vi "WriteRead I2C.vi"(5 "Address":u8, 6 "NoStop (F)":bool, 7 "Bus":u8, 8 "error in (no error)":errorcluster, 9 "Read Len":u8, 10 "Write Data":string, 11 "VISA resource name in":refnum<visa-resource-name>) -> (0 "error out":errorcluster, 1 "Read Data":string, 3 "VISA resource name":refnum<visa-resource-name>)   [LabVIEW 2020, in "CTI-Visa.lvlib"]
uses:
  CTI-Visa.lvlib
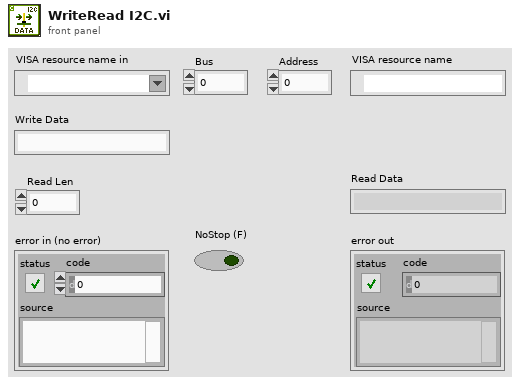
[diagram p1: front panel]
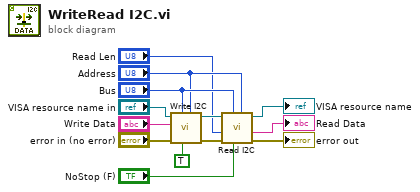
[diagram p0: block diagram]
diagram:
  n1 = call "Write I2C.vi"("Address"="Address", "NoStop (F)"=TRUE, "Bus"="Bus", "error in (no error)"="error in (no error)", "Data"="Write Data", "VISA resource name in"="VISA resource name in") -> ("error out"=w9:errorcluster, "VISA resource name"=w7:refnum<visa-resource-name>)  [unwired: 4 in]
  n2 = call "Read I2C.vi"("Address"="Address", "NoStop (F)"="NoStop (F)", "Bus"="Bus", "error in (no error)"=w9, "Len"="Read Len", "VISA resource name in"=w7) -> ("error out"=→"error out":errorcluster, "Data"=→"Read Data":string, "VISA resource name"=→"VISA resource name":refnum<visa-resource-name>)  [unwired: 3 in]
